vi "CSM DebugTool Dialog.vi"() -> ()   [LabVIEW 2017, in "CSM DebugTool Dialog.lvlib"]
uses:
  CSM DebugTool Dialog.lvlib
  _Shared/CSM Shared.lvlib
panel:
  in  "CSM - Interface Browser":bool
  in  "CSM Mermaid Tool":bool
  in  "CSM State Table Viewer":bool
  in  "CSM State Dashboard":bool
  in  "CSM Debug Console":bool
  in  "CSM Log Viewer":bool
  in  "Owning Application":refnum<vi>
  out "picture":picture
  out "Status":string
  in  "Double Click To Run...":i32(listbox)=-1
  out "Description":string
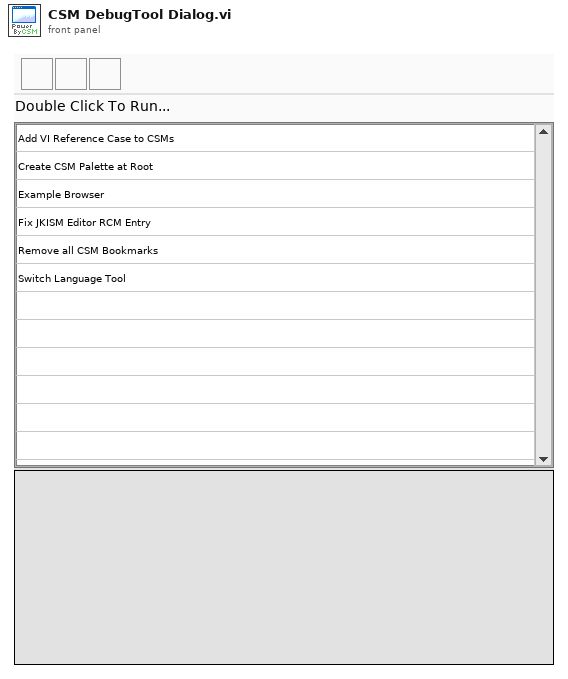
[diagram p1: front panel]
types:
  T1 = enum32{"Invalid", "Standard", "Closed", "Hidden", "Minimized", "Maximized"}
  T2 = enum32{"invalid app kind", "Development System", "Run Time System", "Student Edition", "Embedded LabVIEW", "Evaluation", "Custom"}
  T3 = typedef "LVPoint32TypeDef.ctl" = cluster{"Horizontal":i32, "Vertical":i32}
  T4 = cluster{"Core":cluster{"Current VI Reference":refnum<vi>, "Close Panel on Exit?":bool}, "ToolVIs":path[], "ToolNames":string[]}
  T5 = cluster{"Current VI Reference":refnum<vi>, "Close Panel on Exit?":bool}
  T6 = typedef "imagedata.ctl" = cluster{"image type":i32, "image depth":i32, "image":u8[], "mask":u8[], "colors":u32[], "Rectangle":cluster{"left":i16, "top":i16, "right":i16, "bottom":i16}}
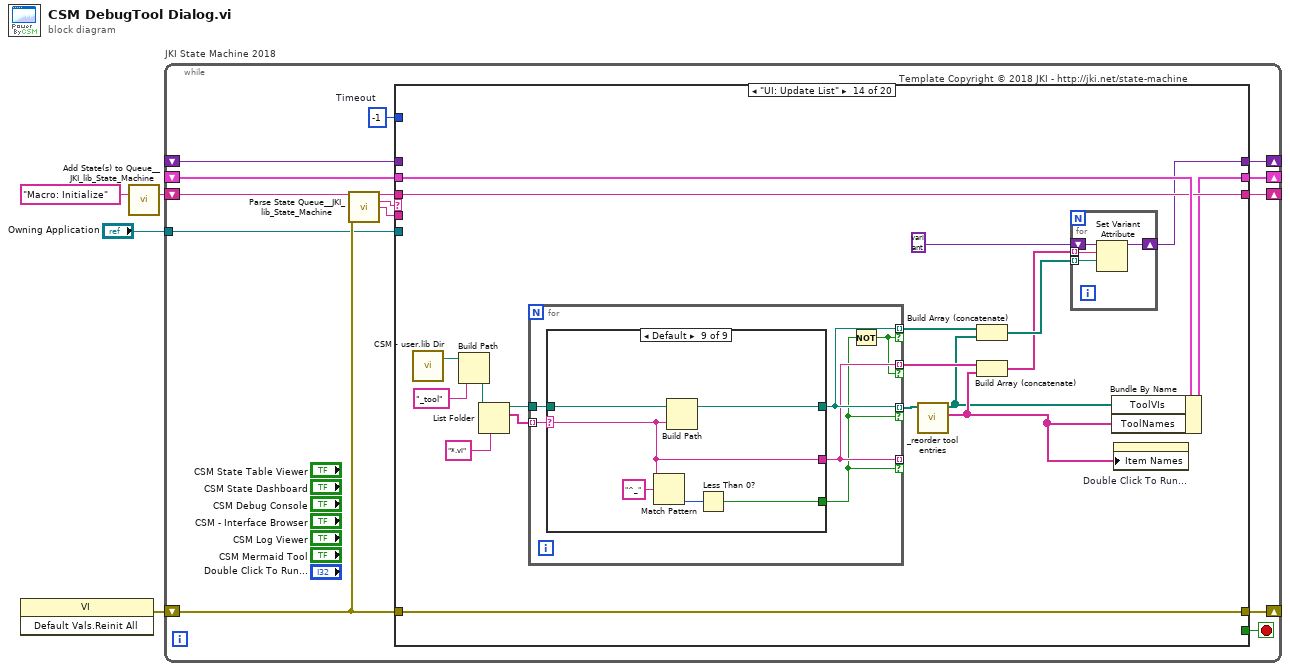
[diagram p0: block diagram]
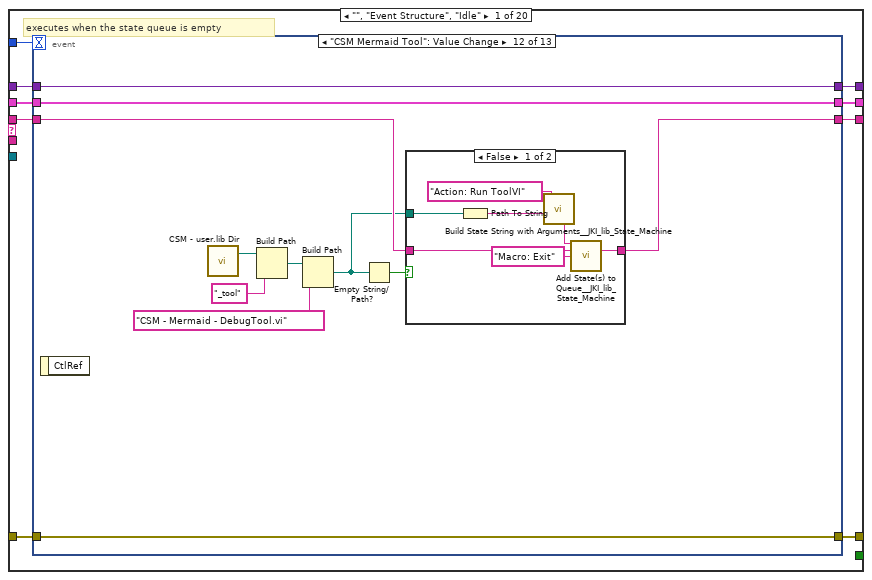
[diagram p2: hidden frame]
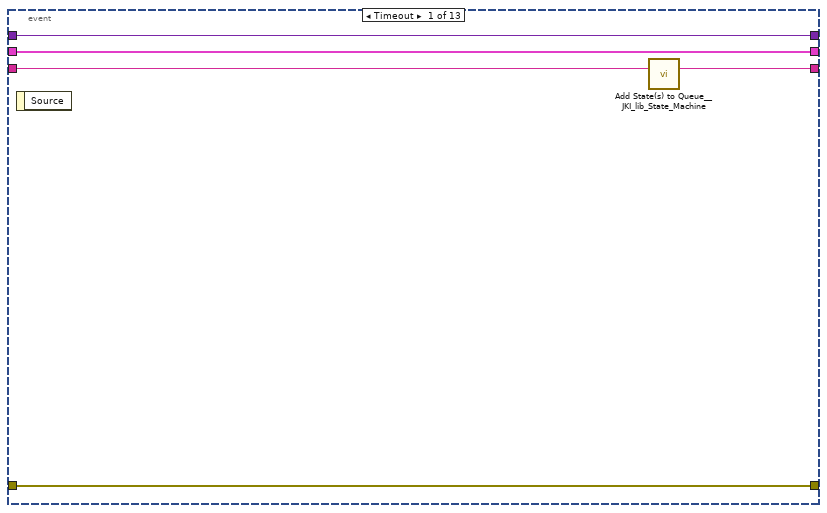
[diagram p3: hidden frame]
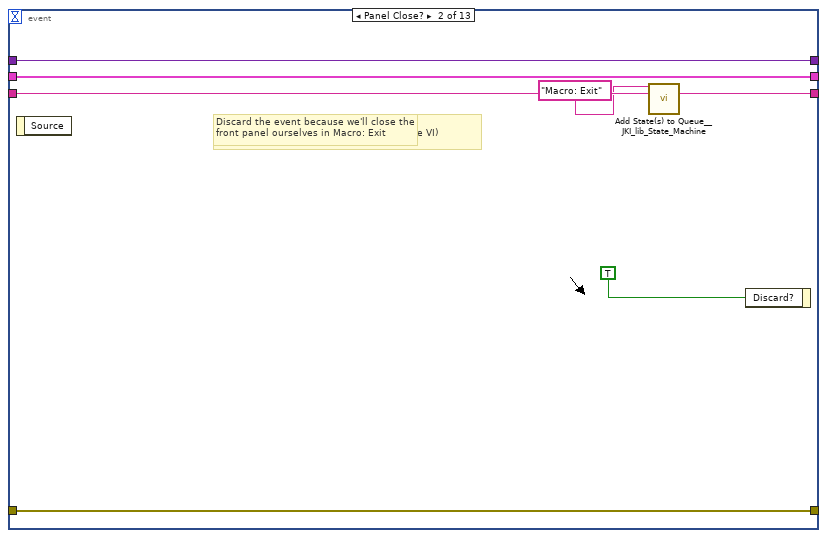
[diagram p4: hidden frame]
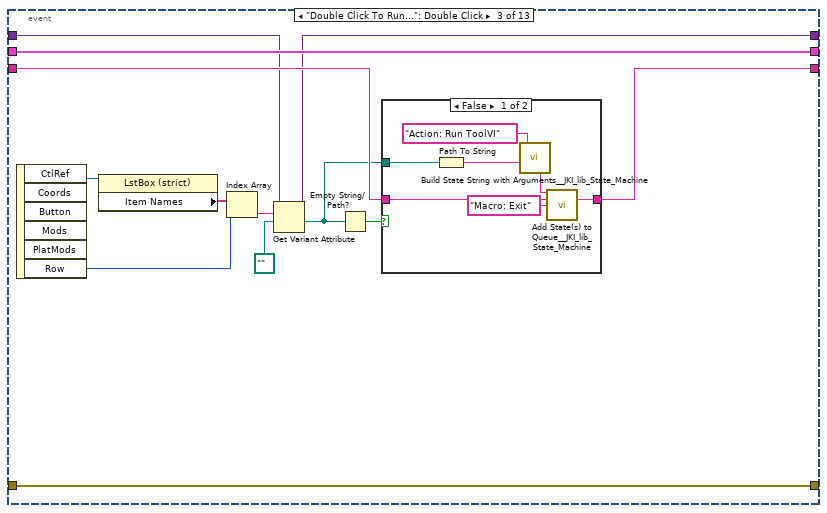
[diagram p5: hidden frame]
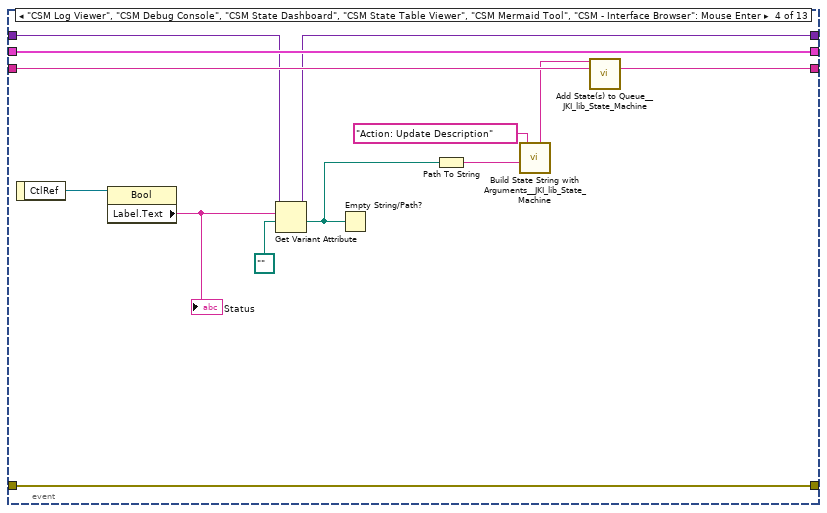
[diagram p7: hidden frame]
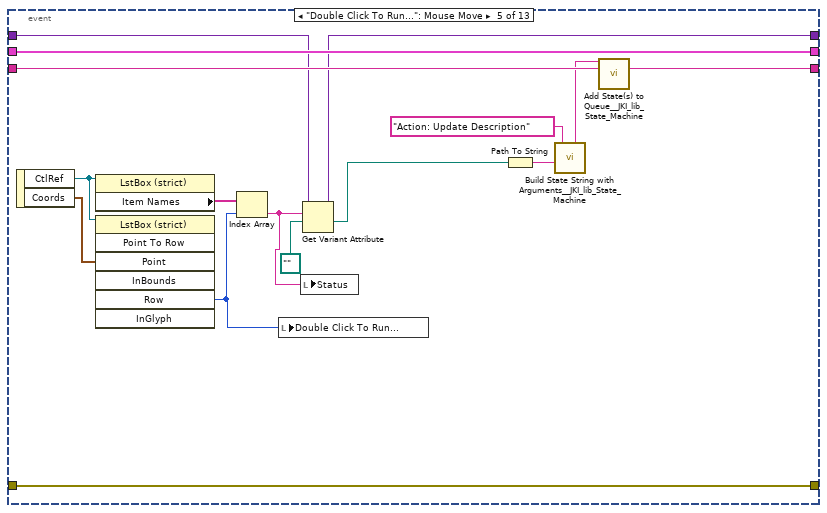
[diagram p8: hidden frame]
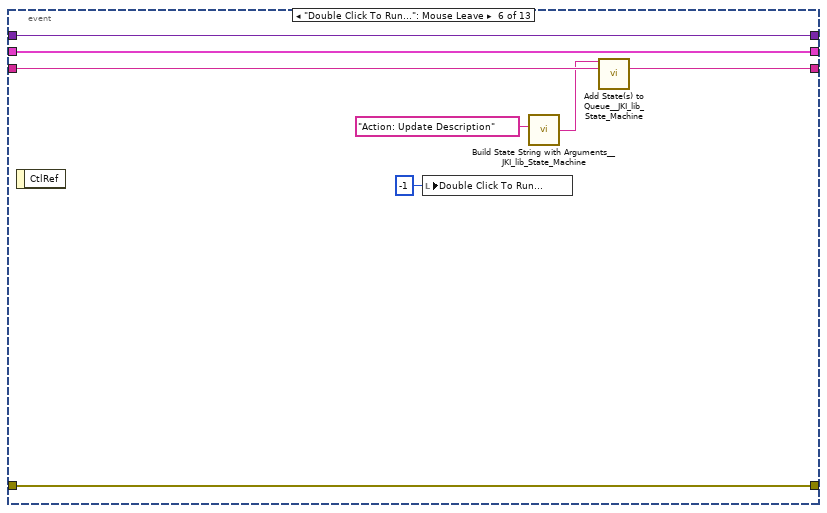
[diagram p9: hidden frame]
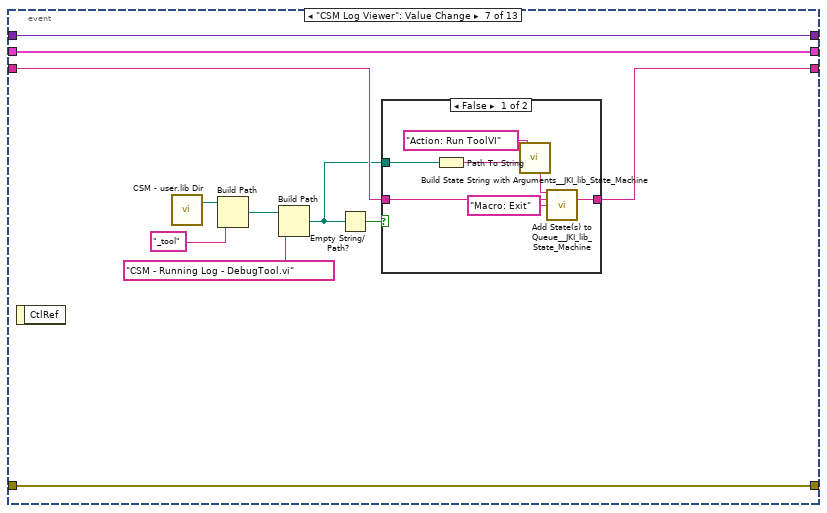
[diagram p10: hidden frame]
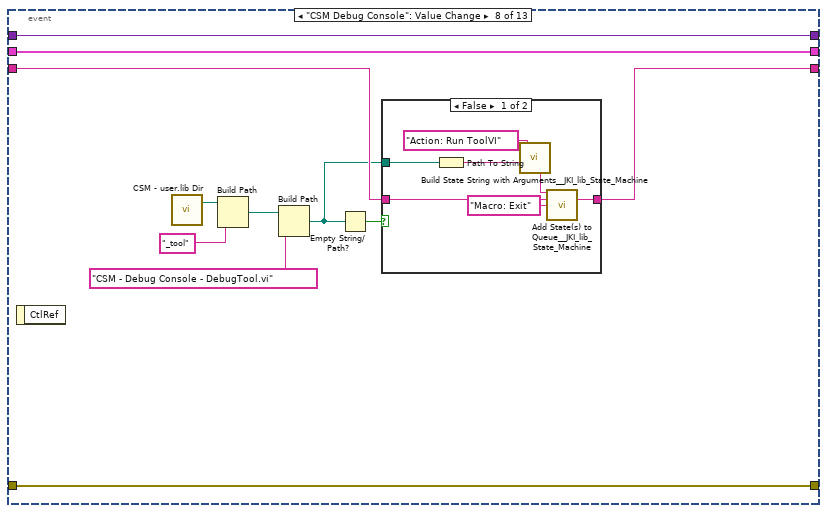
[diagram p12: hidden frame]
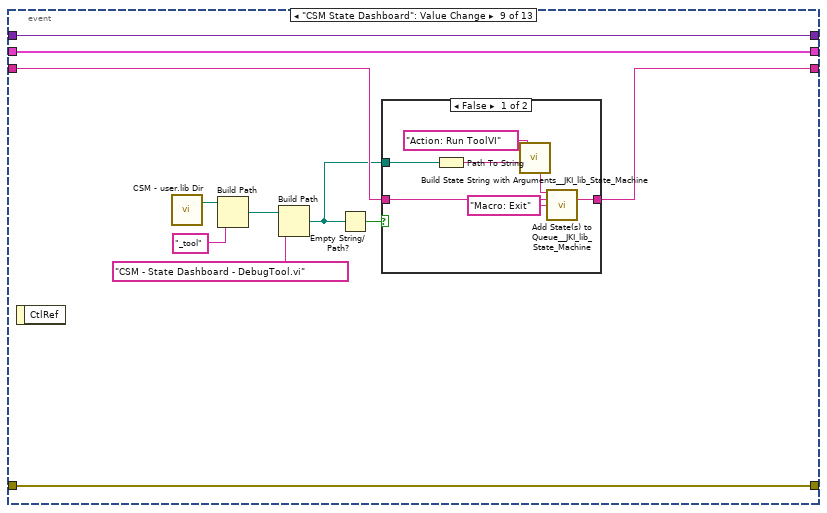
[diagram p14: hidden frame]
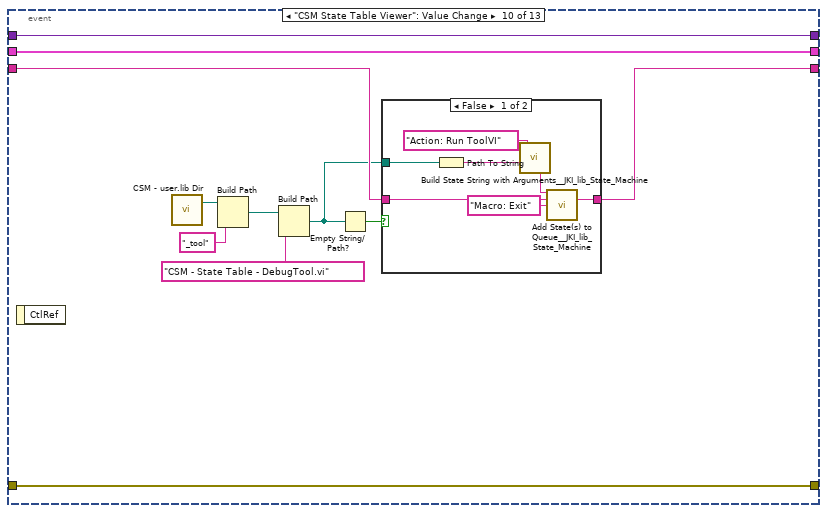
[diagram p16: hidden frame]
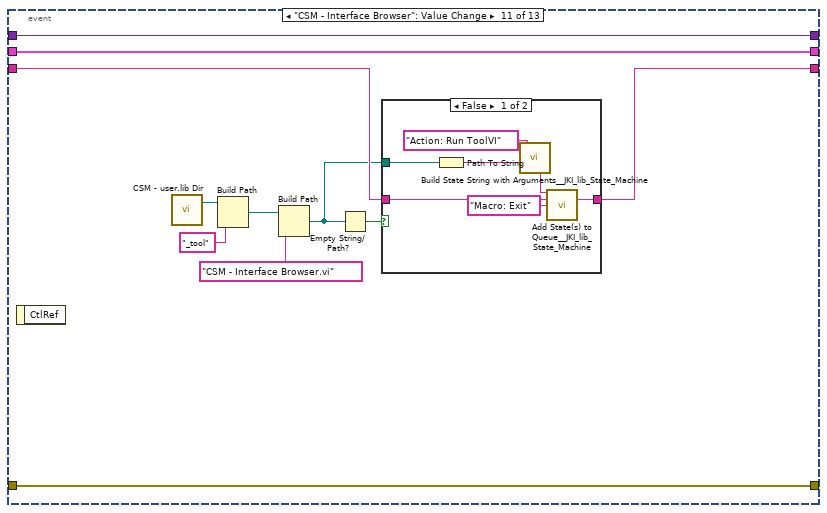
[diagram p18: hidden frame]
diagram:
  n1 = invoke class="VI" method="Default Vals.Reinit All"() -> (error out=w1:errorcluster)  [unwired: 3 in, 2 out]
  n2 = call <vilib>:"Add State(s) to Queue__JKI_lib_State_Machine.vi"("State(s) in (\"\")"="Macro: Initialize") -> ("States Out"=w4:string)  [unwired: 14 in]
  n3 = while "JKI State Machine 2018" {
    shift-right: [w11] -> _
    shift-left: _ -> [w10]
    shift-right: [w14] -> _
    shift-left: w1 -> [w8]
    shift-right: [w13] -> _
    shift-left: w4 -> [w15]
    tunnel: "Owning Application" -> [w7]
    shift-right: [w6] -> _
    shift-left: _ -> [w5]
    stop <- w12 stop-if-true
    w9 = -1  # Timeout
    # "Template Copyright © 2018 JKI - http://jki.net/state-machine"
    n4 = call <vilib>:"Parse State Queue__JKI_lib_State_Machine.vi"("State Queue"=w15, "Error In (no error)"=w8) -> ("Remaining States"=w17:string, "Current State"=w18:string, "Arguments"=w16:string)  [unwired: 11 in]
    n5 = case shown="\"UI: Update List\"" w18 {
      selector: w18 -> [_ _ w223 _ _ _ _ _ _ _ _ _ _ _ _ _ _ _ _ _]
      tunnel: w17 -> [w27 w221 w227 w246 w253 w259 w264 w272 w279 w284 w313 w320 w332 w415 w477 w483 w494 w499 w509 w568]
      tunnel: w16 -> [_ _ _ _ _ _ _ _ _ _ _ w315 w326 _ _ _ _ _ w506 w565]
      tunnel: w10 -> [w25 w218 w225 w240 w250 w257 w261 _ w274 w281 w311 w318 w328 w416 w474 w480 w491 w496 w507 w566]
      tunnel: [w24 w219 w229 _ errorcluster {"status"=FALSE, "code"=0, "source"=""} ("error out") w256 w262 w269 w275 w282 w310 w316 w329 w414 w475 w481 w492 w497 w502 w561] -> w14
      tunnel: w8 -> [w23 w219 w228 _ w249 w256 w262 w269 w276 w282 w310 w317 w330 w414 w475 w481 w492 w497 _ _]
      tunnel: [w26 w220 w226 w245 w252 w258 w263 w271 w278 w283 w312 w319 w331 w415 w476 w482 w493 w498 w508 w567] -> w13
      tunnel: [_ _ _ _ _ TRUE _ _ _ _ _ _ _ _ _ _ _ _ _ _] -> w12
      tunnel: [w22 w218 w225 w244 w250 w257 w261 w270 w274 w281 w311 w318 w328 w410 w474 w480 w491 w496 w507 w566] -> w11
      tunnel: w9 -> [w21 _ _ _ _ _ _ _ _ _ _ _ _ _ _ _ _ _ _ _]
      tunnel: w7 -> [_ _ _ _ _ _ _ _ _ _ _ _ _ _ _ _ _ _ w504 _]
      tunnel: [w20 w217 w222 w235 w247 w254 w260 w265 w273 w280 w309 w314 w325 w405 w473 w478 w484 w495 w501 w564] -> w6
      tunnel: w5 -> [w19 w217 w222 w235 w247 w254 w260 _ w273 w280 w309 w314 w325 _ w473 w478 w484 w495 w501 w564]
      frame "", "Event Structure", "Idle" {
        # "executes when the state queue is empty"
        n6 = event shown="[11] \"CSM Mermaid Tool\": Value Change" {
          selector: _ -> [_ _ _ _ _ _ _ _ _ _ _ _ _]
          dyn-events: _ -> [_ _ _ _ _ _ _ _ _ _ _ _ _]
          timeout: w21 -> [_ _ _ _ _ _ _ _ _ _ _ _ _]
          tunnel: w27 -> [w32 w39 w47 w71 w86 w95 w106 w125 w144 w163 w182 w201 w216]
          tunnel: [w31 w38 w46 w70 w85 w94 w105 w124 w143 w162 w181 w200 w216] -> w26
          tunnel: w25 -> [w29 w36 w49 w72 w87 w96 w107 w126 w145 w164 w183 w202 w214]
          tunnel: [w30 w37 w52 w73 w89 w97 w108 w127 w146 w165 w184 w203 w215] -> w24
          tunnel: w23 -> [w30 w37 w52 w73 w89 w97 w108 w127 w146 w165 w184 w203 w215]
          tunnel: [w29 w36 w49 w72 w87 w96 w107 w126 w145 w164 w183 w202 w214] -> w22
          tunnel: [w28 w33 w43 w68 w83 w92 w101 w120 w139 w158 w177 w196 w213] -> w20
          tunnel: w19 -> [w28 w33 w44 w69 w84 w92 w101 w120 w139 w158 w177 w196 w213]
          event Timeout {
            n7 = event-data() -> ()  [unwired: 1 in, 1 out]
            n8 = call <vilib>:"Add State(s) to Queue__JKI_lib_State_Machine.vi"("State(s) in (\"\")"=w32) -> ("States Out"=w31:string)  [unwired: 14 in]
          }
          event Panel Close? {
            # "Discard the event because we'll close the front panel ourselves in Macro: Exit"
            # "Close Panel button (pressed) Event\n(this executes Macro: Exit to terminate the VI)"
            n9 = event-data() -> ()  [unwired: 1 in, 1 out]
            n10 = call <vilib>:"Add State(s) to Queue__JKI_lib_State_Machine.vi"("State(s) in Front (\"\")"="Macro: Exit", "State(s) in (\"\")"=w39) -> ("States Out"=w38:string)  [unwired: 13 in]
            n11 = event-data("Discard?"=TRUE) -> ()  [unwired: 1 in, 1 out]
          }
          event "Double Click To Run...": Double Click {
            n12 = event-data() -> ("CtlRef"=w51:refnum<vi>, "Row"=w48:i32)  [unwired: 1 in, 4 out]
            n13 = property class="LstBox (strict)"(reference=w51) -> ("Item Names"=w50:string[])  [unwired: 1 in, 2 out]
            n14 = Index Array(array=w50, index=w48) -> (element=w42:string)
            n15 = Get Variant Attribute(Variant=w44, name=w42, default value (empty Variant)=path "") -> (duplicate Variant=w43:variant, value=w40:path)  [unwired: 1 in, 2 out]
            n16 = Empty String/Path?(string/path=w40) -> (empty?=w45:bool)
            n17 = case shown="False" w45 {
              tunnel: w47 -> [w59 w60]
              tunnel: [w58 w60] -> w46
              tunnel: w40 -> [w55 _]
              frame False {
                n18 = Path To String(path=w55) -> (string=w53:string)
                n19 = call <vilib>:"Build State String with Arguments__JKI_lib_State_Machine.vi"("Arguments (\"\")"=w53, "State"="Action: Run ToolVI") -> ("State with Arguments"=w56:string)  [unwired: 4 in]
                n20 = call <vilib>:"Add State(s) to Queue__JKI_lib_State_Machine.vi"("State(s) in Front (\"\")"=w56, "State(s) in (\"\")"=w59, "State(s) at Back (\"\")"="Macro: Exit" ("State(s) at Back (\"\")")) -> ("States Out"=w58:string)  [unwired: 12 in]
              }
              frame True {
              }
            }
          }
          event "CSM Log Viewer", "CSM Debug Console", "CSM State Dashboard", "CSM State Table Viewer", "CSM Mermaid Tool", "CSM - Interface Browser": Mouse Enter {
            n21 = event-data() -> ("CtlRef"=w65:refnum<vi>)  [unwired: 1 in]
            n22 = property class="Bool"(reference=w65) -> ("Label.Text"=w64:string)  [unwired: 1 in, 2 out]
            "Status" <- w64
            n23 = Get Variant Attribute(Variant=w69, name=w64, default value (empty Variant)=path "") -> (duplicate Variant=w68:variant, value=w66:path)  [unwired: 1 in, 2 out]
            n24 = Empty String/Path?(string/path=w66) -> ()  [unwired: 1 out]
            n25 = Path To String(path=w66) -> (string=w61:string)
            n26 = call <vilib>:"Build State String with Arguments__JKI_lib_State_Machine.vi"("Arguments (\"\")"=w61, "State"="Action: Update Description") -> ("State with Arguments"=w63:string)  [unwired: 4 in]
            n27 = call <vilib>:"Add State(s) to Queue__JKI_lib_State_Machine.vi"("State(s) in Front (\"\")"=w63, "State(s) in (\"\")"=w71) -> ("States Out"=w70:string)  [unwired: 13 in]
          }
          event "Double Click To Run...": Mouse Move {
            n28 = event-data() -> ("CtlRef"=w79:refnum<vi>, "Coords"=w80:T3)  [unwired: 1 in]
            n29 = property class="LstBox (strict)"(reference=w79) -> ("Item Names"=w88:string[])  [unwired: 1 in, 2 out]
            n30 = invoke class="LstBox (strict)" method="Point To Row"(reference=w79, "Point"=w80) -> ("Row"=w75:i32)  [unwired: 5 in, 6 out]
            n31 = Index Array(array=w88, index=w75) -> (element=w74:string)
            n32 = local write "Double Click To Run..."(w75) -> ()
            n33 = local write "Status"(w74) -> ()
            n34 = Get Variant Attribute(Variant=w84, name=w74, default value (empty Variant)=path "") -> (duplicate Variant=w83:variant, value=w81:path)  [unwired: 1 in, 2 out]
            n35 = Path To String(path=w81) -> (string=w76:string)
            n36 = call <vilib>:"Build State String with Arguments__JKI_lib_State_Machine.vi"("Arguments (\"\")"=w76, "State"="Action: Update Description") -> ("State with Arguments"=w78:string)  [unwired: 4 in]
            n37 = call <vilib>:"Add State(s) to Queue__JKI_lib_State_Machine.vi"("State(s) in Front (\"\")"=w78, "State(s) in (\"\")"=w86) -> ("States Out"=w85:string)  [unwired: 13 in]
          }
          event "Double Click To Run...": Mouse Leave {
            n38 = event-data() -> ()  [unwired: 1 in, 1 out]
            n39 = local write "Double Click To Run..."(-1 ("Double Click To Run...")) -> ()
            n40 = call <vilib>:"Build State String with Arguments__JKI_lib_State_Machine.vi"("State"="Action: Update Description") -> ("State with Arguments"=w93:string)  [unwired: 5 in]
            n41 = call <vilib>:"Add State(s) to Queue__JKI_lib_State_Machine.vi"("State(s) in Front (\"\")"=w93, "State(s) in (\"\")"=w95) -> ("States Out"=w94:string)  [unwired: 13 in]
          }
          event "CSM Log Viewer": Value Change {
            n42 = event-data() -> ()  [unwired: 1 in, 1 out]
            n43 = call "CSM - user.lib Dir.vi"() -> ("csm_user.lib_dir"=w103:path)  [unwired: 2 in, 1 out]
            n44 = Build Path(base path=w103, name or relative path="_tool") -> (appended path=w100:path)
            n45 = Build Path(base path=w100, name or relative path="CSM - Running Log - DebugTool.vi") -> (appended path=w98:path)
            n46 = Empty String/Path?(string/path=w98) -> (empty?=w104:bool)
            n47 = case shown="False" w104 {
              tunnel: w106 -> [w115 w116]
              tunnel: [w114 w116] -> w105
              tunnel: w98 -> [w111 _]
              frame False {
                n48 = Path To String(path=w111) -> (string=w109:string)
                n49 = call <vilib>:"Build State String with Arguments__JKI_lib_State_Machine.vi"("Arguments (\"\")"=w109, "State"="Action: Run ToolVI") -> ("State with Arguments"=w112:string)  [unwired: 4 in]
                n50 = call <vilib>:"Add State(s) to Queue__JKI_lib_State_Machine.vi"("State(s) in Front (\"\")"=w112, "State(s) in (\"\")"=w115, "State(s) at Back (\"\")"="Macro: Exit" ("State(s) at Back (\"\")")) -> ("States Out"=w114:string)  [unwired: 12 in]
              }
              frame True {
              }
            }
          }
          event "CSM Debug Console": Value Change {
            n51 = event-data() -> ()  [unwired: 1 in, 1 out]
            n52 = call "CSM - user.lib Dir.vi"() -> ("csm_user.lib_dir"=w122:path)  [unwired: 2 in, 1 out]
            n53 = Build Path(base path=w122, name or relative path="_tool") -> (appended path=w119:path)
            n54 = Build Path(base path=w119, name or relative path="CSM - Debug Console - DebugTool.vi") -> (appended path=w117:path)
            n55 = Empty String/Path?(string/path=w117) -> (empty?=w123:bool)
            n56 = case shown="False" w123 {
              tunnel: w125 -> [w134 w135]
              tunnel: [w133 w135] -> w124
              tunnel: w117 -> [w130 _]
              frame False {
                n57 = Path To String(path=w130) -> (string=w128:string)
                n58 = call <vilib>:"Build State String with Arguments__JKI_lib_State_Machine.vi"("Arguments (\"\")"=w128, "State"="Action: Run ToolVI") -> ("State with Arguments"=w131:string)  [unwired: 4 in]
                n59 = call <vilib>:"Add State(s) to Queue__JKI_lib_State_Machine.vi"("State(s) in Front (\"\")"=w131, "State(s) in (\"\")"=w134, "State(s) at Back (\"\")"="Macro: Exit" ("State(s) at Back (\"\")")) -> ("States Out"=w133:string)  [unwired: 12 in]
              }
              frame True {
              }
            }
          }
          event "CSM State Dashboard": Value Change {
            n60 = event-data() -> ()  [unwired: 1 in, 1 out]
            n61 = call "CSM - user.lib Dir.vi"() -> ("csm_user.lib_dir"=w141:path)  [unwired: 2 in, 1 out]
            n62 = Build Path(base path=w141, name or relative path="_tool") -> (appended path=w138:path)
            n63 = Build Path(base path=w138, name or relative path="CSM - State Dashboard - DebugTool.vi") -> (appended path=w136:path)
            n64 = Empty String/Path?(string/path=w136) -> (empty?=w142:bool)
            n65 = case shown="False" w142 {
              tunnel: w144 -> [w153 w154]
              tunnel: [w152 w154] -> w143
              tunnel: w136 -> [w149 _]
              frame False {
                n66 = Path To String(path=w149) -> (string=w147:string)
                n67 = call <vilib>:"Build State String with Arguments__JKI_lib_State_Machine.vi"("Arguments (\"\")"=w147, "State"="Action: Run ToolVI") -> ("State with Arguments"=w150:string)  [unwired: 4 in]
                n68 = call <vilib>:"Add State(s) to Queue__JKI_lib_State_Machine.vi"("State(s) in Front (\"\")"=w150, "State(s) in (\"\")"=w153, "State(s) at Back (\"\")"="Macro: Exit" ("State(s) at Back (\"\")")) -> ("States Out"=w152:string)  [unwired: 12 in]
              }
              frame True {
              }
            }
          }
          event "CSM State Table Viewer": Value Change {
            n69 = event-data() -> ()  [unwired: 1 in, 1 out]
            n70 = call "CSM - user.lib Dir.vi"() -> ("csm_user.lib_dir"=w160:path)  [unwired: 2 in, 1 out]
            n71 = Build Path(base path=w160, name or relative path="_tool") -> (appended path=w157:path)
            n72 = Build Path(base path=w157, name or relative path="CSM - State Table - DebugTool.vi") -> (appended path=w155:path)
            n73 = Empty String/Path?(string/path=w155) -> (empty?=w161:bool)
            n74 = case shown="False" w161 {
              tunnel: w163 -> [w172 w173]
              tunnel: [w171 w173] -> w162
              tunnel: w155 -> [w168 _]
              frame False {
                n75 = Path To String(path=w168) -> (string=w166:string)
                n76 = call <vilib>:"Build State String with Arguments__JKI_lib_State_Machine.vi"("Arguments (\"\")"=w166, "State"="Action: Run ToolVI") -> ("State with Arguments"=w169:string)  [unwired: 4 in]
                n77 = call <vilib>:"Add State(s) to Queue__JKI_lib_State_Machine.vi"("State(s) in Front (\"\")"=w169, "State(s) in (\"\")"=w172, "State(s) at Back (\"\")"="Macro: Exit" ("State(s) at Back (\"\")")) -> ("States Out"=w171:string)  [unwired: 12 in]
              }
              frame True {
              }
            }
          }
          event "CSM - Interface Browser": Value Change {
            n78 = event-data() -> ()  [unwired: 1 in, 1 out]
            n79 = call "CSM - user.lib Dir.vi"() -> ("csm_user.lib_dir"=w179:path)  [unwired: 2 in, 1 out]
            n80 = Build Path(base path=w179, name or relative path="_tool") -> (appended path=w176:path)
            n81 = Build Path(base path=w176, name or relative path="CSM - Interface Browser.vi") -> (appended path=w174:path)
            n82 = Empty String/Path?(string/path=w174) -> (empty?=w180:bool)
            n83 = case shown="False" w180 {
              tunnel: w182 -> [w191 w192]
              tunnel: [w190 w192] -> w181
              tunnel: w174 -> [w187 _]
              frame False {
                n84 = Path To String(path=w187) -> (string=w185:string)
                n85 = call <vilib>:"Build State String with Arguments__JKI_lib_State_Machine.vi"("Arguments (\"\")"=w185, "State"="Action: Run ToolVI") -> ("State with Arguments"=w188:string)  [unwired: 4 in]
                n86 = call <vilib>:"Add State(s) to Queue__JKI_lib_State_Machine.vi"("State(s) in Front (\"\")"=w188, "State(s) in (\"\")"=w191, "State(s) at Back (\"\")"="Macro: Exit" ("State(s) at Back (\"\")")) -> ("States Out"=w190:string)  [unwired: 12 in]
              }
              frame True {
              }
            }
          }
          event "CSM Mermaid Tool": Value Change {
            n87 = event-data() -> ()  [unwired: 1 in, 1 out]
            n88 = call "CSM - user.lib Dir.vi"() -> ("csm_user.lib_dir"=w198:path)  [unwired: 2 in, 1 out]
            n89 = Build Path(base path=w198, name or relative path="_tool") -> (appended path=w195:path)
            n90 = Build Path(base path=w195, name or relative path="CSM - Mermaid - DebugTool.vi") -> (appended path=w193:path)
            n91 = Empty String/Path?(string/path=w193) -> (empty?=w199:bool)
            n92 = case shown="False" w199 {
              tunnel: w201 -> [w210 w211]
              tunnel: [w209 w211] -> w200
              tunnel: w193 -> [w206 _]
              frame False {
                n93 = Path To String(path=w206) -> (string=w204:string)
                n94 = call <vilib>:"Build State String with Arguments__JKI_lib_State_Machine.vi"("Arguments (\"\")"=w204, "State"="Action: Run ToolVI") -> ("State with Arguments"=w207:string)  [unwired: 4 in]
                n95 = call <vilib>:"Add State(s) to Queue__JKI_lib_State_Machine.vi"("State(s) in Front (\"\")"=w207, "State(s) in (\"\")"=w210, "State(s) at Back (\"\")"="Macro: Exit" ("State(s) at Back (\"\")")) -> ("States Out"=w209:string)  [unwired: 12 in]
              }
              frame True {
              }
            }
          }
          event "CSM Log Viewer", "CSM Debug Console", "CSM State Dashboard", "CSM State Table Viewer", "CSM Mermaid Tool", "CSM - Interface Browser": Mouse Leave {
            n96 = event-data() -> ()  [unwired: 1 in, 4 out]
            n97 = local write "Status"("" ("Status 2")) -> ()
          }
        }
      }
      frame "---------- Core ----------" {
        # "Do not put any code in this frame.\n(it is a separator no-op)"
        n98 = call <vilib>:"Add State(s) to Queue__JKI_lib_State_Machine.vi"("State(s) in (\"\")"=w221) -> ("States Out"=w220:string)  [unwired: 14 in]
      }
      frame Default {
        w232 = 42 items=["No error", "Argument error", "Memory is full", "Out of zone", "End of file", "File already open", "Generic file I/O error", "File not found", "File permission error", "Disk is full", "Duplicate path", "Too many files open", "System feature not enabled", "Resource file not found", "Cannot add resource", "Resource not found", "Image not found", "Image memory error", "Pen does not exist", "Config type invalid", "Config token not found", "Config parse error", "Config memory error", "Bad external code format", "Bad external code offset", "External code not present", "Null window", "Destroy window error", "Null menu", "Print aborted", "Bad print record", "Print driver error", "Windows error during printing", "Memory error during printing", "Print dialog error", "Generic print error", "Invalid device refnum", "Device not found", "Device parameter error", "Device unit error", "Cannot open device", "Device call aborted", "Generic error", "Cancelled by user", "Object ID too low", "Object ID too high", "Object not in heap", "Unknown heap", "Unknown object (invalid DefProc)", "Unknown object (DefProc not in table)", "Message out of range", "Invalid (null) method", "Unknown message", "Manager call not supported", "Bad address", "Network operation in progress", "Network operation timed out", "Connection is busy", "Network attribute not supported", "Network error", "Address in use", "System out of memory", "Connection aborted", "Connection refused", "Not connected", "Already connected", "Connection closed", "Initialization error (interapplication manager)", "Bad occurrence", "Wait on unbound occurrence handler", "Occurrence queue overflow", "Datalog type conflict", "Unused", "Unrecognized type (interapplication manager)", "Memory corrupt", "Failed to make temporary DLL", "Old CIN version", "Drag socket not found", "Failed to load drop-object", "Failed to register OLE object", "Failed to release OLE object", "Format specifier type mismatch", "Unknown format specifier", "Too few format specifiers", "Too many format specifiers", "Scan failed", "Newer CIN version", "Error converting to variant", "Runtime menu error", "Password tampered", "Variant attribute not found", "Incompatible variant data type", "Event data is not available", "Event Store is not present", "Occurrence is not found", "Event Queue is not created", "Event info is not available", "Refnum passed is NULL", "Error retrieving Class GUID", "Error retrieving CoClass GUID", "Error retrieving TypeLib GUID.", "Bad built application magic bytes.", "Specific driver is different from the specific driver associated with the Logical Name.", "There is no session opened to the class driver.", "Max Error", "MAX - Error with config objects", "MAX - Error loading configuration", "MAX - Group not supported"]
        # "Current State"
        # "Do not delete, rename, or modify this frame.\n(this is used to capture unhandled states and typos)"
        # "Handle mistyped state name (developer tool)"
        n99 = Format Into String(format string="Software Exception: Unhandled State \"%s\"." ("message"), error in=w228, w223) -> (resulting string=w231:string, error out=w230:errorcluster)  [unwired: 1 in]
        n100 = call <vilib>:"Error Cluster From Error Code.vi"("show call chain? (False)"=TRUE, "error in (no error)"=w230, "error message (\"\")"=w231, "error code (0)"=w232) -> ("error out"=w229:errorcluster)  [unwired: 5 in]
        n101 = call <vilib>:"Add State(s) to Queue__JKI_lib_State_Machine.vi"("State(s) in (\"\")"=w227) -> ("States Out"=w226:string)  [unwired: 14 in]
      }
      frame "Initialize Core Data" {
        # "Do not delete, rename, or modify this frame.\n(this is used to determine panel behavior on exit)"
        # "originally closed?"
        # "exe?"
        # "If panel starts closed or is an EXE, then close it when we exit"
        n102 = property class="VI"() -> ("FP.State"=w238:T1)  [unwired: 2 in, 2 out]
        n103 = property class="App"() -> ("App.Kind"=w243:T2)  [unwired: 2 in, 2 out]
        n104 = control-ref of="Current VI Reference"() -> (w234:refnum<vi>)
        n105 = Equal?(x=w238, y=T1."Closed" ("Front Panel Window:State")) -> (x = y?=w236:bool)
        n106 = Equal?(x=w243, y=T2."Run Time System" ("Application:Kind")) -> (x = y?=w241:bool)
        n107 = Or(x=w236, y=w241) -> (x .or. y?=w239:bool)
        n108 = call "CSM DebugTool Dialog Ref(FGV).vi"("VI Reference"=w234) -> ()  [unwired: 10 in, 1 out]
        n109 = Bundle By Name(cluster=w240, "Core.Current VI Reference"=w234, "Core.Close Panel on Exit?"=w239) -> (w244:T4)
        n110 = call <vilib>:"Add State(s) to Queue__JKI_lib_State_Machine.vi"("State(s) in (\"\")"=w246) -> ("States Out"=w245:string)  [unwired: 14 in]
      }
      frame "Error Handler" {
        # "Unhandled Error -- Display it"
        # "Handle any errors here.\nYou can also output any states to clean-up after errors occur"
        # "Clear error"
        n111 = call <vilib>:"General Error Handler.vi"("error in (no error)"=w249) -> ()  [unwired: 10 in, 5 out]
        n112 = call <vilib>:"Add State(s) to Queue__JKI_lib_State_Machine.vi"("State(s) in Front (\"\")"="/* Post Error States", "State(s) in (\"\")"=w253) -> ("States Out"=w252:string)  [unwired: 13 in]
      }
      frame "Exit" {
        # "Do not put any code in this frame.\n(No errors that occur here will be handled.)"
        n113 = call <vilib>:"Add State(s) to Queue__JKI_lib_State_Machine.vi"("State(s) in (\"\")"=w259) -> ("States Out"=w258:string)  [unwired: 14 in]
      }
      frame "---------- Data ----------" {
        # "Do not put any code in this frame.\n(It is a separator no-op. You can make a copy of this frame to create a new Data frame)"
        n114 = call <vilib>:"Add State(s) to Queue__JKI_lib_State_Machine.vi"("State(s) in (\"\")"=w264) -> ("States Out"=w263:string)  [unwired: 14 in]
      }
      frame "Data: Initialize" {
        w266 = string[] []  # ToolNames
        w267 = path[] []  # ToolVIs
        w268 = T5 {"Current VI Reference"=refnum, "Close Panel on Exit?"=FALSE}  # Core
        w265 = variant  # Tool Name-Path Map
        # "do not delete - used by framework"
        # "Initialize the shift-register data, here.\n(data names are defined by what you wire into the bundle function)"
        n115 = Bundle("Core"=w268, "ToolVIs"=w267, "ToolNames"=w266) -> (w270:T4)  [unwired: 1 in]
        n116 = call <vilib>:"Add State(s) to Queue__JKI_lib_State_Machine.vi"("State(s) in (\"\")"=w272) -> ("States Out"=w271:string)  [unwired: 14 in]
      }
      frame "Data: Cleanup" {
        # "Cleanup any data and references, here.\n(this is called automatically, by the Macro: Exit)"
        n117 = Unbundle By Name(w274) -> ("Core.Current VI Reference"=w277:refnum<vi>)
        n118 = Close Reference(reference=w277, error in (no error)=w276) -> (error out=w275:errorcluster)
        n119 = call <vilib>:"Add State(s) to Queue__JKI_lib_State_Machine.vi"("State(s) in (\"\")"=w279) -> ("States Out"=w278:string)  [unwired: 14 in]
      }
      frame "---------- UI ----------" {
        # "Do not put any code in this frame.\n(It is a separator no-op. You can make a copy of this frame to create a new UI frame)"
        n120 = call <vilib>:"Add State(s) to Queue__JKI_lib_State_Machine.vi"("State(s) in (\"\")"=w284) -> ("States Out"=w283:string)  [unwired: 14 in]
      }
      frame "UI: Initialize" {
        # "Initialize the User Interface, here.\n(this is called automatically, by the Macro: Init)"
        n121 = call "CSM - user.lib Dir.vi"() -> ("csm_user.lib_dir"=w307:path)  [unwired: 2 in, 1 out]
        n122 = Build Path(base path=w307, name or relative path="_tool") -> (appended path=w285:path)
        n123 = Build Path(base path=w285, name or relative path="CSM - State Table - DebugTool.vi") -> (appended path=w290:path)
        n124 = Build Path(base path=w285, name or relative path="CSM - Mermaid - DebugTool.vi") -> (appended path=w304:path)
        n125 = Build Path(base path=w285, name or relative path="CSM - State Dashboard - DebugTool.vi") -> (appended path=w295:path)
        n126 = call <vilib>:"Check if File or Folder Exists.vi"("path"=w290) -> ("error out"=w288:errorcluster, "file or folder exists?"=w287:bool)  [unwired: 8 in, 1 out]
        n127 = call <vilib>:"Check if File or Folder Exists.vi"("path"=w304) -> ("error out"=w302:errorcluster, "file or folder exists?"=w301:bool)  [unwired: 8 in, 1 out]
        n128 = call <vilib>:"Check if File or Folder Exists.vi"("path"=w295) -> ("error out"=w297:errorcluster, "file or folder exists?"=w298:bool)  [unwired: 8 in, 1 out]
        n129 = Not(x=w288) -> (.not. x?=w286:bool)
        n130 = Not(x=w302) -> (.not. x?=w300:bool)
        n131 = Not(x=w297) -> (.not. x?=w299:bool)
        n132 = control-ref of="CSM State Table Viewer"() -> (w292:refnum<vi>)
        n133 = control-ref of="CSM Mermaid Tool"() -> (w308:refnum<vi>)
        n134 = control-ref of="CSM State Dashboard"() -> (w293:refnum<vi>)
        n135 = And(x=w287, y=w286) -> (x .and. y?=w289:bool)
        n136 = And(x=w301, y=w300) -> (x .and. y?=w303:bool)
        n137 = And(x=w298, y=w299) -> (x .and. y?=w296:bool)
        n138 = property class="Bool"(reference=w292, "Visible"=w289) -> ()  [unwired: 1 in, 2 out]
        n139 = property class="Bool"(reference=w308, "Visible"=w303) -> ()  [unwired: 1 in, 2 out]
        n140 = property class="Bool"(reference=w293, "Visible"=w296) -> ()  [unwired: 1 in, 2 out]
        n141 = call <vilib>:"Add State(s) to Queue__JKI_lib_State_Machine.vi"("State(s) in (\"\")"=w313) -> ("States Out"=w312:string)  [unwired: 14 in]
      }
      frame "UI: Cursor Set" {
        # "Argument"
        # "Set and Unset Cursor Busy.\n(Usage: \"UI: Cursor Set >> Busy|Idle\")"
        n142 = case shown="\"Busy\"" w315 {
          tunnel: w317 -> [w322 w324]
          tunnel: [w321 w323] -> w316
          frame "Idle", Default {
            n143 = call <vilib>:"Unset Busy.vi"("error in (no error)"=w322) -> ("error out"=w321:errorcluster)  [unwired: 10 in]
          }
          frame "Busy" {
            n144 = call <vilib>:"Set Busy.vi"("error in (no error)"=w324) -> ("error out"=w323:errorcluster)  [unwired: 9 in, 1 out]
          }
        }
        n145 = call <vilib>:"Add State(s) to Queue__JKI_lib_State_Machine.vi"("State(s) in (\"\")"=w320) -> ("States Out"=w319:string)  [unwired: 14 in]
      }
      frame "UI: Front Panel State" {
        # "Argument"
        # "Set Front Panel Open or Closed\n(Usage: \"UI: Front Panel State >> Open|Close\")"
        n146 = Unbundle By Name(w328) -> ("Core.Current VI Reference"=w327:refnum<vi>)
        n147 = case shown="\"Minimize\", \"Minimized\"" w326 {
          tunnel: w330 -> [w338 w353 w364 w377 w390]
          tunnel: [w340 w354 w366 w379 w392] -> w329
          tunnel: w327 -> [w339 w351 w365 w378 w391]
          frame "Open", "Standard", Default {
            w333 = T1."Standard" ("State")
            n148 = property class="VI"(reference=w339, error in=w338) -> (reference out=w336:refnum<vi>, error out=w337:errorcluster, "FP.State"=w335:T1)
            n149 = Not Equal?(x=w335, y=w333) -> (x != y?=w334:bool)
            n150 = case shown="True" w334 {
              tunnel: [w344 w346] -> w340
              tunnel: w337 -> [w343 w346]
              tunnel: w336 -> [w342 _]
              tunnel: w333 -> [w341 _]
              frame True {
                n151 = invoke class="VI" method="FP.Open"(reference=w342, error in=w343, "Activate"=TRUE, "State"=w341) -> (error out=w344:errorcluster)  [unwired: 1 in, 4 out]
              }
              frame False {
              }
            }
          }
          frame "Close", "Closed" {
            n152 = property class="VI"(reference=w351, error in=w353) -> (reference out=w350:refnum<vi>, error out=w352:errorcluster, "FP.State"=w348:T1)
            n153 = Not Equal?(x=w348, y=T1."Closed" ("Front Panel Window:State")) -> (x != y?=w347:bool)
            n154 = case shown="True" w347 {
              tunnel: [w355 w358] -> w354
              tunnel: w352 -> [w355 w357]
              tunnel: w350 -> [_ w356]
              frame False {
              }
              frame True {
                n155 = invoke class="VI" method="FP.Close"(reference=w356, error in=w357) -> (error out=w358:errorcluster)  [unwired: 1 in, 2 out]
              }
            }
          }
          frame "Hidden", "Hide" {
            w359 = T1."Hidden" ("State")
            n156 = property class="VI"(reference=w365, error in=w364) -> (reference out=w362:refnum<vi>, error out=w363:errorcluster, "FP.State"=w361:T1)
            n157 = Not Equal?(x=w361, y=w359) -> (x != y?=w360:bool)
            n158 = case shown="True" w360 {
              tunnel: [w370 w371] -> w366
              tunnel: w363 -> [w369 w371]
              tunnel: w362 -> [w368 _]
              tunnel: w359 -> [w367 _]
              frame True {
                n159 = invoke class="VI" method="FP.Open"(reference=w368, error in=w369, "State"=w367) -> (error out=w370:errorcluster)  [unwired: 2 in, 4 out]
              }
              frame False {
              }
            }
          }
          frame "Minimize", "Minimized" {
            w372 = T1."Minimized" ("State")
            n160 = property class="VI"(reference=w378, error in=w377) -> (reference out=w375:refnum<vi>, error out=w376:errorcluster, "FP.State"=w374:T1)
            n161 = Not Equal?(x=w374, y=w372) -> (x != y?=w373:bool)
            n162 = case shown="True" w373 {
              tunnel: [w383 w384] -> w379
              tunnel: w376 -> [w382 w384]
              tunnel: w375 -> [w381 _]
              tunnel: w372 -> [w380 _]
              frame True {
                n163 = invoke class="VI" method="FP.Open"(reference=w381, error in=w382, "State"=w380) -> (error out=w383:errorcluster)  [unwired: 2 in, 4 out]
              }
              frame False {
              }
            }
          }
          frame "Maximize", "Maximized" {
            w385 = T1."Maximized" ("State")
            n164 = property class="VI"(reference=w391, error in=w390) -> (reference out=w388:refnum<vi>, error out=w389:errorcluster, "FP.State"=w387:T1)
            n165 = Not Equal?(x=w387, y=w385) -> (x != y?=w386:bool)
            n166 = case shown="True" w386 {
              tunnel: [w396 w397] -> w392
              tunnel: w389 -> [w395 w397]
              tunnel: w388 -> [w394 _]
              tunnel: w385 -> [w393 _]
              frame True {
                n167 = invoke class="VI" method="FP.Open"(reference=w394, error in=w395, "State"=w393) -> (error out=w396:errorcluster)  [unwired: 2 in, 4 out]
              }
              frame False {
              }
            }
          }
        }
        n168 = call <vilib>:"Add State(s) to Queue__JKI_lib_State_Machine.vi"("State(s) in (\"\")"=w332) -> ("States Out"=w331:string)  [unwired: 14 in]
      }
      frame "UI: Update List" {
        n169 = call "CSM - user.lib Dir.vi"() -> ("csm_user.lib_dir"=w409:path)  [unwired: 2 in, 1 out]
        n170 = Build Path(base path=w409, name or relative path="_tool") -> (appended path=w408:path)
        n171 = List Folder(path=w408, pattern="*.vi") -> (path out=w411:path, filenames=w412:string[])  [unwired: 2 in, 2 out]
        n172 = for {
          tunnel: w412 -> [w425] mode=indexing
          tunnel: w411 -> [w426]
          tunnel: [w424] -> w400 mode=indexing if=w422
          tunnel: [w423] -> _ mode=indexing if=w422
          tunnel: [w424] -> w403 mode=indexing if=w421
          tunnel: [w423] -> w404 mode=indexing if=w421
          n173 = case shown="Default" w425 {
            selector: w425 -> [w427 w432 w437 w442 w447 w452 w457 w462 w467]
            tunnel: w426 -> [w431 w436 w441 w446 w451 w456 w461 w466 w471]
            tunnel: [FALSE FALSE FALSE FALSE FALSE FALSE TRUE TRUE w469] -> w422
            tunnel: [w428 w433 w438 w443 w448 w453 w458 w463 w468] -> w424
            tunnel: ["CSM Log Viewer" "CSM Debug Console" "CSM - Interface Browser" "CSM Mermaid Tool" "CSM State Dashboard" "CSM State Table Viewer" "Switch CSM Language Support..." "Refresh More Template palette..." w467] -> w423
            frame "CSM - Running Log - DebugTool.vi" {
              n174 = Build Path(base path=w431, name or relative path=w427) -> (appended path=w428:path)
            }
            frame "CSM - Debug Console - DebugTool.vi" {
              n175 = Build Path(base path=w436, name or relative path=w432) -> (appended path=w433:path)
            }
            frame "CSM - Interface Browser.vi" {
              n176 = Build Path(base path=w441, name or relative path=w437) -> (appended path=w438:path)
            }
            frame "CSM - Mermaid - DebugTool.vi" {
              n177 = Build Path(base path=w446, name or relative path=w442) -> (appended path=w443:path)
            }
            frame "CSM - State Dashboard - DebugTool.vi" {
              n178 = Build Path(base path=w451, name or relative path=w447) -> (appended path=w448:path)
            }
            frame "CSM - State Table - DebugTool.vi" {
              n179 = Build Path(base path=w456, name or relative path=w452) -> (appended path=w453:path)
            }
            frame "CSM - Switch Language Tool.vi" {
              n180 = Build Path(base path=w461, name or relative path=w457) -> (appended path=w458:path)
            }
            frame "CSM - Refesh More Template Palette.vi" {
              n181 = Build Path(base path=w466, name or relative path=w462) -> (appended path=w463:path)
            }
            frame Default {
              n182 = Match Pattern(string=w467, regular expression="^_") -> (offset past match=w470:i32)  [unwired: 1 in, 3 out]
              n183 = Build Path(base path=w471, name or relative path=w467) -> (appended path=w468:path)
              n184 = Less Than 0?(x=w470) -> (x < 0?=w469:bool)
            }
          }
          n185 = Not(x=w422) -> (.not. x?=w421:bool)
        }
        n186 = call "_reorder tool entries.vi"("Path Control"=w400) -> ("After"=w399:string[], "Path Control (dup)"=w398:path[])  [unwired: 9 in]
        n187 = Build Array (concatenate)(w403, w398) -> (w402:path[])
        n188 = Build Array (concatenate)(w404, w399) -> (w401:string[])
        n189 = for {
          shift-right: [w420] -> w405
          shift-left: variant -> [w419]
          tunnel: w401 -> [w418] mode=indexing
          tunnel: w402 -> [w417] mode=indexing
          n190 = Set Variant Attribute(Variant=w419, name=w418, value=w417) -> (Variant out=w420:variant)  [unwired: 1 in, 2 out]
        }
        n191 = Bundle By Name(cluster=w416, "ToolVIs"=w398, "ToolNames"=w399) -> (w410:T4)
        n192 = property on="Double Click To Run..." class="LstBox (strict)"("Item Names"=w399) -> ()  [unwired: 2 in, 2 out]
      }
      frame "---------- Macro ----------" {
        # "Do not put any code in this frame.\n(It is a separator no-op. You can make a copy of this frame to create a new Macro frame)"
        n193 = call <vilib>:"Add State(s) to Queue__JKI_lib_State_Machine.vi"("State(s) in (\"\")"=w477) -> ("States Out"=w476:string)  [unwired: 14 in]
      }
      frame "Macro: Initialize" {
        w479 = "Data: Initialize\nInitialize Core Data\nUI: Initialize\nUI: Front Panel State >> Open\nUI: Update List"  # Data: Initialize Initialize Core Data UI: Initialize UI: Front Panel State >> Open UI: Update List
        # "Initialization Macro\n(This is called once, when the VI starts)"
        n194 = call <vilib>:"Add State(s) to Queue__JKI_lib_State_Machine.vi"("State(s) in Front (\"\")"=w479, "State(s) in (\"\")"=w483) -> ("States Out"=w482:string)  [unwired: 13 in]
      }
      frame "Macro: Exit" {
        # "Exit Macro\n(This is called once, when the VI exits)"
        n195 = Unbundle By Name(w491) -> ("Core.Close Panel on Exit?"=w490:bool)
        n196 = Select(t="UI: Front Panel State >> Close", s=w490, f="") -> (s? t:f=w487:string)
        n197 = call <vilib>:"Add State(s) to Queue__JKI_lib_State_Machine.vi"("State(s) in (\"\")"=w487, "State(s) at Back (\"\")"="Data: Cleanup\nExit") -> ("States Out"=w485:string)  [unwired: 13 in]
        n198 = call <vilib>:"Add State(s) to Queue__JKI_lib_State_Machine.vi"("State(s) in Front (\"\")"=w485, "State(s) in (\"\")"=w494) -> ("States Out"=w493:string)  [unwired: 13 in]
      }
      frame "---------- Action ----------" {
        # "Template Separator\n(You can make a copy of, or modify, this frame)"
        n199 = call <vilib>:"Add State(s) to Queue__JKI_lib_State_Machine.vi"("State(s) in (\"\")"=w499) -> ("States Out"=w498:string)  [unwired: 14 in]
      }
      frame "Action: Run ToolVI" {
        # "Your code here.\n(You can make a copy of, or modify, this frame)"
        n200 = String To Path(string=w506) -> (path=w505:path)
        n201 = Not A Number/Path/Refnum?(number/path/refnum=w504) -> (NaN/Path/Refnum?=w503:bool)
        n202 = while {
          tunnel: w505 -> [w518]
          tunnel: w504 -> [w517]
          tunnel: w503 -> [w516]
          shift-right: [w511] -> w502
          shift-left: errorcluster {"status"=FALSE, "code"=0, "source"=""} ("error out") -> [w513]
          i -> [w515]
          stop <- w512 stop-if-true
          n203 = case shown="0" w515 {
            tunnel: w518 -> [_ w524 w544]
            tunnel: w517 -> [_ w523 w543]
            tunnel: w516 -> [_ w522 w542]
            tunnel: [w519 w521 w541] -> w511
            tunnel: [TRUE _ _] -> w514
            tunnel: w513 -> [w519 _ _]
            frame Default {
            }
            frame 0 {
              n204 = case shown="True" w522 {
                tunnel: [w532 w538] -> w526
                tunnel: [w531 w537] -> w525
                tunnel: w524 -> [w529 w535]
                tunnel: w523 -> [_ w534]
                frame True {
                  n205 = Open VI Reference(type specifier VI Refnum (for type only)=refnum<vi> refnum, vi path=w529, options=128) -> (vi reference=w532:refnum<vi>, error out=w531:errorcluster)  [unwired: 3 in]
                }
                frame False {
                  n206 = Open VI Reference(type specifier VI Refnum (for type only)=refnum<vi> refnum, application reference (local)=w534, vi path=w535, options=128) -> (vi reference=w538:refnum<vi>, error out=w537:errorcluster)  [unwired: 2 in]
                }
              }
              n207 = call-by-ref "Start Asynchronous Call"(reference=w526, error in=w525) -> (reference out=w528:refnum<vi>, error out=w527:errorcluster)  [unwired: 12 in]
              n208 = Close Reference(reference=w528, error in (no error)=w527) -> (error out=w521:errorcluster)
            }
            frame 1 {
              n209 = case shown="False" w542 {
                tunnel: [w552 w558] -> w546
                tunnel: [w551 w557] -> w545
                tunnel: w544 -> [w550 w556]
                tunnel: w543 -> [_ w555]
                tunnel: refnum<vi> refnum ("type specifier VI Refnum (for type only)") -> [w549 w554]
                frame True {
                  n210 = Open VI Reference(type specifier VI Refnum (for type only)=w549, vi path=w550, options=128) -> (vi reference=w552:refnum<vi>, error out=w551:errorcluster)  [unwired: 3 in]
                }
                frame False {
                  n211 = Open VI Reference(type specifier VI Refnum (for type only)=w554, application reference (local)=w555, vi path=w556, options=128) -> (vi reference=w558:refnum<vi>, error out=w557:errorcluster)  [unwired: 2 in]
                }
              }
              n212 = call-by-ref "Start Asynchronous Call"(reference=w546, error in=w545) -> (reference out=w548:refnum<vi>, error out=w547:errorcluster)  [unwired: 12 in]
              n213 = Close Reference(reference=w548, error in (no error)=w547) -> (error out=w541:errorcluster)
            }
          }
          n214 = Not(x=w511) -> (.not. x?=w510:bool)
          n215 = Or(x=w510, y=w514) -> (x .or. y?=w512:bool)
        }
        n216 = call <vilib>:"Add State(s) to Queue__JKI_lib_State_Machine.vi"("State(s) in (\"\")"=w509) -> ("States Out"=w508:string)  [unwired: 14 in]
      }
      frame "Action: Update Description" {
        # "Your code here.\n(You can make a copy of, or modify, this frame)"
        n217 = case shown="Default" w565 {
          selector: w565 -> [_ w578]
          tunnel: [_ w573] -> w563
          tunnel: [_ w577] -> w562
          tunnel: [_ w570] -> w560
          frame "" {
          }
          frame Default {
            n218 = String To Path(string=w578) -> (path=w569:path)
            n219 = invoke class="App" method="Get VI.Description"("VI Path"=w569) -> (error out=w577:errorcluster, "VI Desc"=w574:string)  [unwired: 4 in, 3 out]
            n220 = invoke class="App" method="Get VI.Title"("VI Path"=w569) -> ("VI Title"=w575:string)  [unwired: 4 in, 4 out]
            n221 = invoke class="App" method="Get VI.Icon"("Path"=w569) -> ("Get VI.Icon"=w572:T6)  [unwired: 3 in, 3 out]
            n222 = call <vilib>:"Draw Flattened Pixmap.vi"("image data"=w572, "picture"=picture data[5B]) -> ("new picture"=w570:picture)  [unwired: 7 in]
            n223 = Empty String/Path?(string/path=w574) -> (empty?=w576:bool)
            n224 = Select(t=w575, s=w576, f=w574) -> (s? t:f=w573:string)
          }
        }
        "Description" <- w563
        "picture" <- w560
        n225 = call <vilib>:"Clear Errors.vi"("error in (no error)"=w562) -> ("error out"=w561:errorcluster)  [unwired: 5 in, 1 out]
        n226 = call <vilib>:"Add State(s) to Queue__JKI_lib_State_Machine.vi"("State(s) in (\"\")"=w568) -> ("States Out"=w567:string)  [unwired: 14 in]
      }
    }
  }
